vi "FinalSystem.vi"() -> ()   [LabVIEW 2017]
panel:
  in  "stop":bool
  out "Countdown":dbl
  out "x .or. y?":bool
  out "Frequency":dbl
  out "Ambulance":bool
  out "Fire":bool
  out "Police":bool
  out "Waveform Graph":dynamicdata(graph)
  out "Velocity":dbl
  out "Too Fast":bool
  out "Delta T":dbl
  out "Elapsed Time (s)":dbl
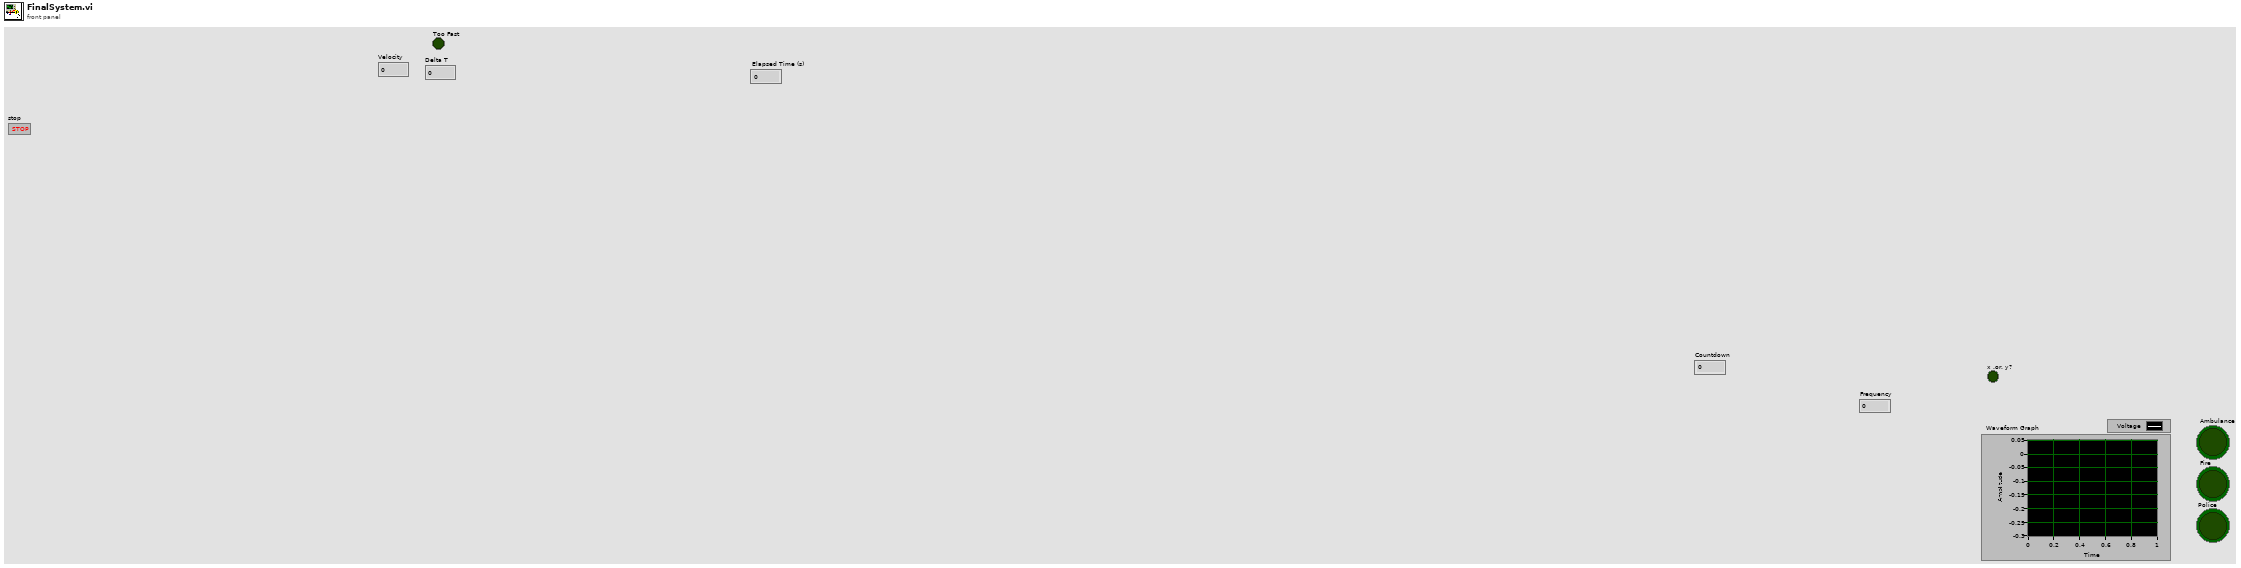
[diagram p1: front panel]
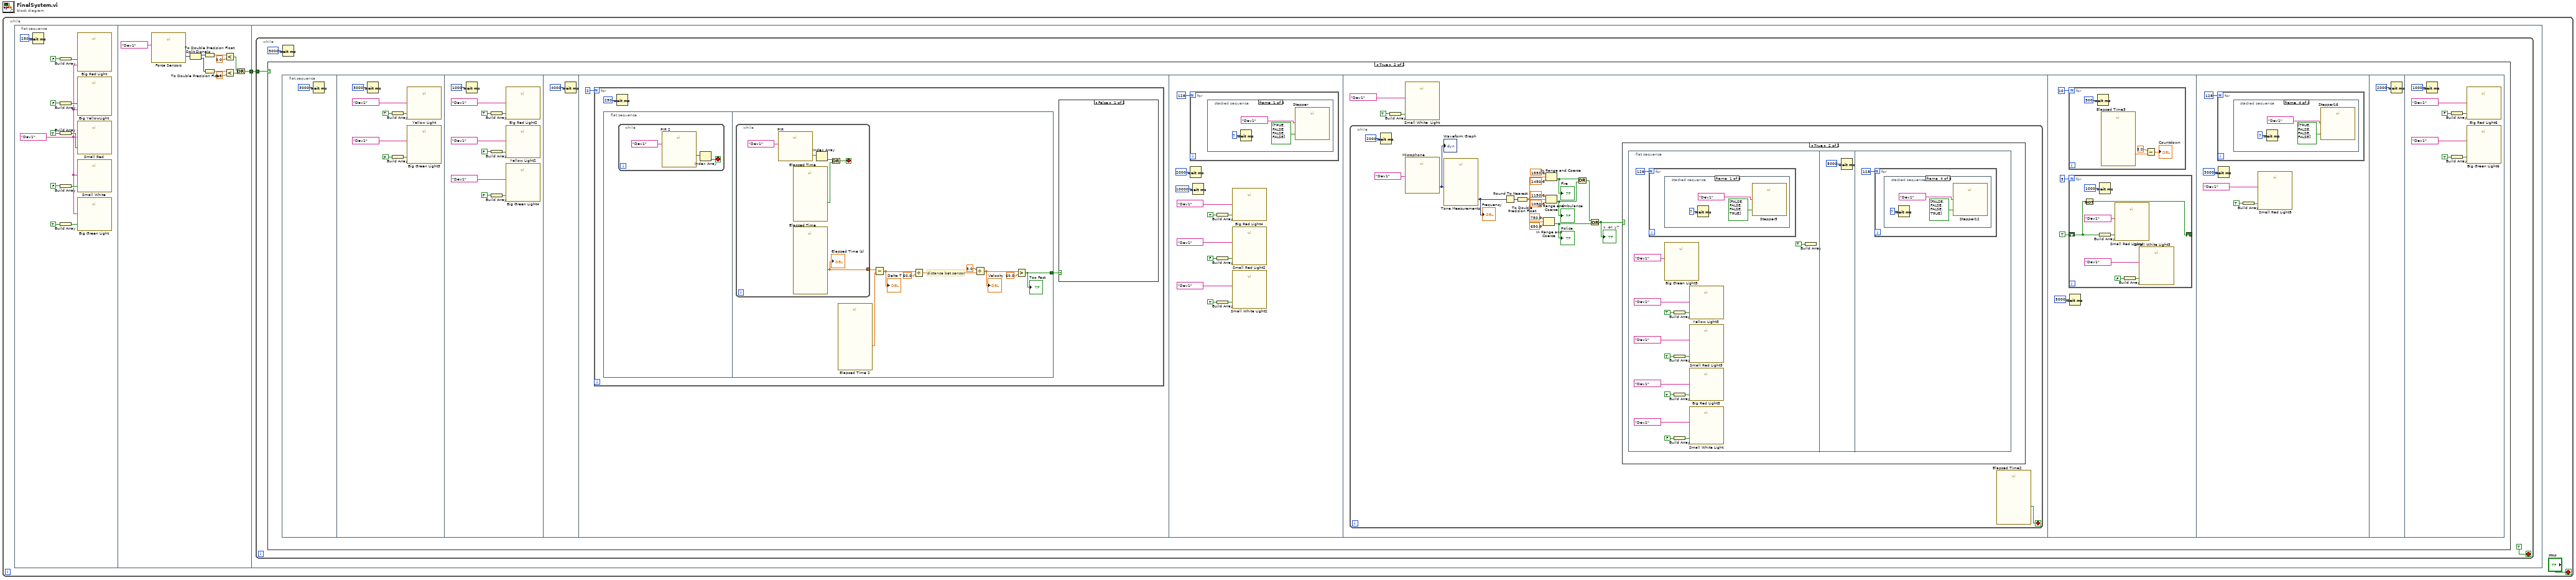
[diagram p0: block diagram]
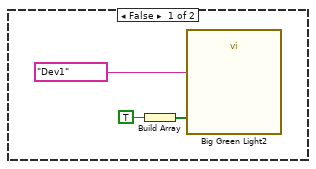
[diagram p2: hidden frame]
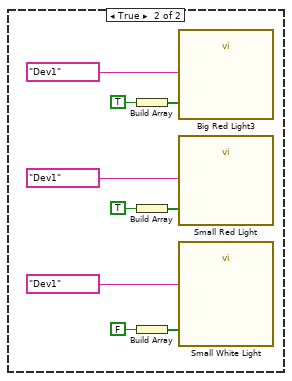
[diagram p3: hidden frame]
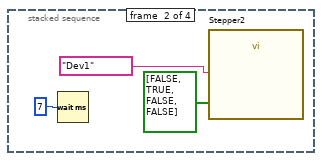
[diagram p4: hidden frame]
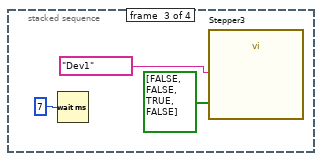
[diagram p5: hidden frame]
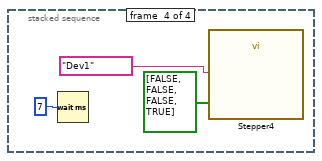
[diagram p6: hidden frame]
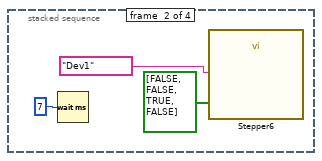
[diagram p8: hidden frame]
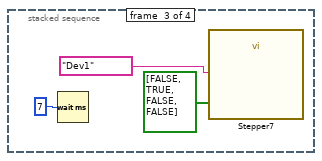
[diagram p9: hidden frame]
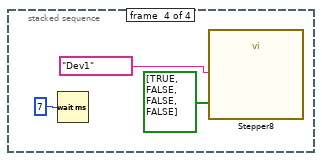
[diagram p10: hidden frame]
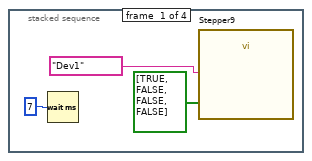
[diagram p11: hidden frame]
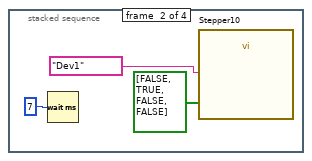
[diagram p12: hidden frame]
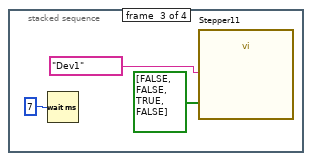
[diagram p13: hidden frame]
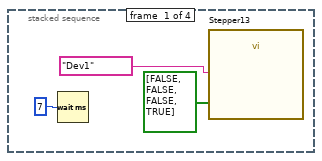
[diagram p14: hidden frame]
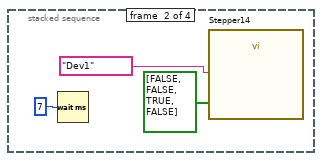
[diagram p15: hidden frame]
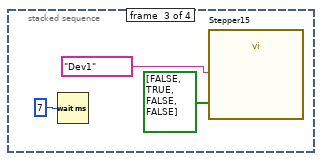
[diagram p16: hidden frame]
diagram:
  n1 = while {
    stop <- "stop" stop-if-true
    n2 = flat-sequence {
      tunnel: [w15] -> w2
      tunnel: w2 -> [w26]
      frame #0 {
        w3 = tag "Dev1" ("device name")
        n3 = Wait (ms)(milliseconds to wait=u32 250) -> ()  [unwired: 1 out]
        n4 = Build Array(FALSE) -> (w12:bool[])
        n5 = Build Array(FALSE) -> (w10:bool[])
        n6 = Build Array(TRUE) -> (w8:bool[])
        n7 = Build Array(FALSE) -> (w6:bool[])
        n8 = Build Array(TRUE) -> (w14:bool[])
        n9 = call "Big Red Light"("data"=w12, "device name"=w3) -> ()  [unwired: 16 in, 2 out]
        n10 = call "Big YellowLight"("data"=w10, "device name"=w3) -> ()  [unwired: 16 in, 2 out]
        n11 = call "Small Red"("data"=w8, "device name"=w3) -> ()  [unwired: 16 in, 2 out]
        n12 = call "Small White"("data"=w6, "device name"=w3) -> ()  [unwired: 16 in, 2 out]
        n13 = call "Big Green Light"("data"=w14, "device name"=w3) -> ()  [unwired: 16 in, 2 out]
      }
      frame #1 {
        n14 = call "Force Sensors"("device name"=tag "Dev1") -> ("data"=w18:dynamicdata)  [unwired: 16 in, 2 out]
        n15 = Split Signals(w18) -> (w17:dynamicdata, w16:dynamicdata)  [unwired: 2 in]
        n16 = To Double Precision Float(number=w17) -> (double precision float=w25:dbl)
        n17 = To Double Precision Float(number=w16) -> (double precision float=w22:dbl)
        n18 = Less?(x=w25, y=3.0) -> (x < y?=w19:bool)
        n19 = Less?(x=w22, y=3.0) -> (x < y?=w20:bool)
        n20 = Or(x=w19, y=w20) -> (x .or. y?=w15:bool)
      }
      frame #2 {
        n21 = while {
          tunnel: w26 -> [w28]
          stop <- TRUE stop-if-true
          n22 = case shown="True" w28 {
            frame False {
              n23 = Build Array(TRUE) -> (w32:bool[])
              n24 = call "Big Green Light2"("data"=w32, "device name"=tag "Dev1") -> ()  [unwired: 16 in, 2 out]
            }
            frame True {
              n25 = flat-sequence {
                frame #0 {
                  n26 = Wait (ms)(milliseconds to wait=u32 3000) -> ()  [unwired: 1 out]
                }
                frame #1 {
                  n27 = Wait (ms)(milliseconds to wait=u32 3000) -> ()  [unwired: 1 out]
                  n28 = Build Array(TRUE) -> (w40:bool[])
                  n29 = Build Array(FALSE) -> (w34:bool[])
                  n30 = call "Yellow Light"("data"=w40, "device name"=tag "Dev1") -> ()  [unwired: 16 in, 2 out]
                  n31 = call "Big Green Light3"("data"=w34, "device name"=tag "Dev1") -> ()  [unwired: 16 in, 2 out]
                }
                frame #2 {
                  n32 = Wait (ms)(milliseconds to wait=u32 1000) -> ()  [unwired: 1 out]
                  n33 = Build Array(TRUE) -> (w50:bool[])
                  n34 = Build Array(FALSE) -> (w49:bool[])
                  n35 = Build Array(FALSE) -> (w41:bool[])
                  n36 = call "Big Red Light2"("data"=w50, "device name"=tag "Dev1") -> ()  [unwired: 16 in, 2 out]
                  n37 = call "Yellow Light2"("data"=w49, "device name"=tag "Dev1") -> ()  [unwired: 16 in, 2 out]
                  n38 = call "Big Green Light4"("data"=w41, "device name"=tag "Dev1") -> ()  [unwired: 16 in, 2 out]
                }
                frame #3 {
                  n39 = Wait (ms)(milliseconds to wait=u32 4000) -> ()  [unwired: 1 out]
                }
                frame #4 {
                  n40 = for {
                    N: 2 -> [_]
                    n41 = flat-sequence {
                      tunnel: [w59] -> w53
                      frame #0 {
                        n42 = while {
                          stop <- w56 stop-if-true
                          n43 = call "PIR 2"("device name"=tag "Dev1") -> ("data"=w57:bool[])  [unwired: 16 in, 2 out]
                          n44 = Index Array(array=w57) -> (element=w56:bool)  [unwired: 1 in]
                        }
                      }
                      frame #1 {
                        # "distance bet sensor"
                        n45 = while {
                          tunnel: [w71] -> w61
                          stop <- w67 stop-if-true
                          n46 = call "PIR"("device name"=tag "Dev1") -> ("data"=w72:bool[])  [unwired: 16 in, 2 out]
                          n47 = call "Elapsed Time"() -> ("Time has Elapsed"=w68:bool)  [unwired: 12 in, 7 out]
                          n48 = call "Elapsed Time"() -> ("Elapsed Time (s)"=w71:dbl)  [unwired: 12 in, 7 out]
                          "Elapsed Time (s)" <- w71
                          n49 = Index Array(array=w72) -> (element=w69:bool)  [unwired: 1 in]
                          n50 = Or(x=w69, y=w68) -> (x .or. y?=w67:bool)
                        }
                        n51 = call "Elapsed Time 2"() -> ("Elapsed Time (s)"=w58:dbl)  [unwired: 12 in, 7 out]
                        n52 = Subtract(x=w61, y=w58) -> (x-y=w60:dbl)
                        "Delta T" <- w60
                        n53 = Divide(x=w60, y=60.0) -> (x/y=w63:dbl)
                        n54 = Divide(x=5.0, y=w63) -> (x/y=w65:dbl)
                        "Velocity" <- w65
                        n55 = Greater?(x=w65, y=60.0) -> (0:w59:bool)
                        "Too Fast" <- w59
                      }
                    }
                    n56 = Wait (ms)(milliseconds to wait=u32 250) -> ()  [unwired: 1 out]
                    n57 = case shown="False" w53 {
                      frame False {
                      }
                      frame True {
                        n58 = Build Array(TRUE) -> (w79:bool[])
                        n59 = Build Array(TRUE) -> (w80:bool[])
                        n60 = Build Array(FALSE) -> (w81:bool[])
                        n61 = call "Big Red Light3"("data"=w79, "device name"=tag "Dev1") -> ()  [unwired: 16 in, 2 out]
                        n62 = call "Small Red Light"("data"=w80, "device name"=tag "Dev1") -> ()  [unwired: 16 in, 2 out]
                        n63 = call "Small White Light"("data"=w81, "device name"=tag "Dev1") -> ()  [unwired: 16 in, 2 out]
                      }
                    }
                  }
                }
                frame #5 {
                  n64 = for {
                    N: 128 -> [_]
                    n65 = stacked-sequence {
                      frame #0 {
                        n66 = Wait (ms)(milliseconds to wait=u32 7) -> ()  [unwired: 1 out]
                        n67 = call "Stepper"("data"=bool[] [TRUE, FALSE, FALSE, FALSE], "device name"=tag "Dev1") -> ()  [unwired: 16 in, 2 out]
                      }
                      frame #1 {
                        n68 = Wait (ms)(milliseconds to wait=u32 7) -> ()  [unwired: 1 out]
                        n69 = call "Stepper2"("data"=bool[] [FALSE, TRUE, FALSE, FALSE], "device name"=tag "Dev1") -> ()  [unwired: 16 in, 2 out]
                      }
                      frame #2 {
                        n70 = Wait (ms)(milliseconds to wait=u32 7) -> ()  [unwired: 1 out]
                        n71 = call "Stepper3"("data"=bool[] [FALSE, FALSE, TRUE, FALSE], "device name"=tag "Dev1") -> ()  [unwired: 16 in, 2 out]
                      }
                      frame #3 {
                        n72 = Wait (ms)(milliseconds to wait=u32 7) -> ()  [unwired: 1 out]
                        n73 = call "Stepper4"("data"=bool[] [FALSE, FALSE, FALSE, TRUE], "device name"=tag "Dev1") -> ()  [unwired: 16 in, 2 out]
                      }
                    }
                  }
                  n74 = Wait (ms)(milliseconds to wait=u32 2000) -> ()  [unwired: 1 out]
                  n75 = Wait (ms)(milliseconds to wait=u32 10000) -> ()  [unwired: 1 out]
                  n76 = Build Array(TRUE) -> (w86:bool[])
                  n77 = Build Array(FALSE) -> (w91:bool[])
                  n78 = Build Array(TRUE) -> (w87:bool[])
                  n79 = call "Big Red Light4"("data"=w86, "device name"=tag "Dev1") -> ()  [unwired: 16 in, 2 out]
                  n80 = call "Small Red Light2"("data"=w91, "device name"=tag "Dev1") -> ()  [unwired: 16 in, 2 out]
                  n81 = call "Small White Light2"("data"=w87, "device name"=tag "Dev1") -> ()  [unwired: 16 in, 2 out]
                }
                frame #6 {
                  n82 = while {
                    stop <- w109 stop-if-true
                    n83 = Wait (ms)(milliseconds to wait=u32 2000) -> ()  [unwired: 1 out]
                    n84 = call "Microphone"("device name"=tag "Dev1") -> ("data"=w126:dynamicdata)  [unwired: 16 in, 2 out]
                    "Waveform Graph" <- w126
                    n85 = call "Tone Measurements"("Signals"=w126) -> ("Frequency"=w112:dynamicdata)  [unwired: 8 in, 2 out]
                    "Frequency" <- w112
                    n86 = Round To Nearest(number=w112) -> (nearest integer value=w111:dynamicdata)
                    n87 = To Double Precision Float(number=w111) -> (double precision float=w119:dbl)
                    n88 = In Range and Coerce(upper limit=750.0 ("y"), x=w119, lower limit=650.0 ("y")) -> (In Range?=w115:bool)  [unwired: 1 out]
                    "Police" <- w115
                    n89 = In Range and Coerce(upper limit=1550.0 ("y"), x=w119, lower limit=1450.0 ("y")) -> (In Range?=w117:bool)  [unwired: 1 out]
                    "Fire" <- w117
                    n90 = In Range and Coerce(upper limit=1150.0 ("y"), x=w119, lower limit=1050.0 ("y")) -> (In Range?=w116:bool)  [unwired: 1 out]
                    "Ambulance" <- w116
                    n91 = Or(x=w117, y=w116) -> (x .or. y?=w118:bool)
                    n92 = Or(x=w118, y=w115) -> (x .or. y?=w110:bool)
                    "x .or. y?" <- w110
                    n93 = case shown="True" w110 {
                      frame False {
                      }
                      frame True {
                        n94 = flat-sequence {
                          frame #0 {
                            n95 = for {
                              N: 128 -> [_]
                              n96 = stacked-sequence {
                                frame #0 {
                                n97 = Wait (ms)(milliseconds to wait=u32 7) -> ()  [unwired: 1 out]
                                n98 = call "Stepper5"("data"=bool[] [FALSE, FALSE, FALSE, TRUE], "device name"=tag "Dev1") -> ()  [unwired: 16 in, 2 out]
                                }
                                frame #1 {
                                n99 = Wait (ms)(milliseconds to wait=u32 7) -> ()  [unwired: 1 out]
                                n100 = call "Stepper6"("data"=bool[] [FALSE, FALSE, TRUE, FALSE], "device name"=tag "Dev1") -> ()  [unwired: 16 in, 2 out]
                                }
                                frame #2 {
                                n101 = Wait (ms)(milliseconds to wait=u32 7) -> ()  [unwired: 1 out]
                                n102 = call "Stepper7"("data"=bool[] [FALSE, TRUE, FALSE, FALSE], "device name"=tag "Dev1") -> ()  [unwired: 16 in, 2 out]
                                }
                                frame #3 {
                                n103 = Wait (ms)(milliseconds to wait=u32 7) -> ()  [unwired: 1 out]
                                n104 = call "Stepper8"("data"=bool[] [TRUE, FALSE, FALSE, FALSE], "device name"=tag "Dev1") -> ()  [unwired: 16 in, 2 out]
                                }
                              }
                            }
                            n105 = call "Big Green Light5"("device name"=tag "Dev1") -> ()  [unwired: 17 in, 2 out]
                            n106 = Build Array(TRUE) -> (w140:bool[])
                            n107 = Build Array(TRUE) -> (w130:bool[])
                            n108 = Build Array(TRUE) -> (w141:bool[])
                            n109 = Build Array(FALSE) -> (w127:bool[])
                            n110 = call "Yellow Light3"("data"=w140, "device name"=tag "Dev1") -> ()  [unwired: 16 in, 2 out]
                            n111 = call "Small Red Light3"("data"=w130, "device name"=tag "Dev1") -> ()  [unwired: 16 in, 2 out]
                            n112 = call "Big Red Light5"("data"=w141, "device name"=tag "Dev1") -> ()  [unwired: 16 in, 2 out]
                            n113 = call "Small White Light"("data"=w127, "device name"=tag "Dev1") -> ()  [unwired: 16 in, 2 out]
                            n114 = Build Array(TRUE) -> ()  [unwired: 1 out]
                          }
                          frame #1 {
                            n115 = Wait (ms)(milliseconds to wait=u32 5000) -> ()  [unwired: 1 out]
                          }
                          frame #2 {
                            n116 = for {
                              N: 128 -> [_]
                              n117 = stacked-sequence {
                                frame #0 {
                                n118 = Wait (ms)(milliseconds to wait=u32 7) -> ()  [unwired: 1 out]
                                n119 = call "Stepper9"("data"=bool[] [TRUE, FALSE, FALSE, FALSE], "device name"=tag "Dev1") -> ()  [unwired: 16 in, 2 out]
                                }
                                frame #1 {
                                n120 = Wait (ms)(milliseconds to wait=u32 7) -> ()  [unwired: 1 out]
                                n121 = call "Stepper10"("data"=bool[] [FALSE, TRUE, FALSE, FALSE], "device name"=tag "Dev1") -> ()  [unwired: 16 in, 2 out]
                                }
                                frame #2 {
                                n122 = Wait (ms)(milliseconds to wait=u32 7) -> ()  [unwired: 1 out]
                                n123 = call "Stepper11"("data"=bool[] [FALSE, FALSE, TRUE, FALSE], "device name"=tag "Dev1") -> ()  [unwired: 16 in, 2 out]
                                }
                                frame #3 {
                                n124 = Wait (ms)(milliseconds to wait=u32 7) -> ()  [unwired: 1 out]
                                n125 = call "Stepper12"("data"=bool[] [FALSE, FALSE, FALSE, TRUE], "device name"=tag "Dev1") -> ()  [unwired: 16 in, 2 out]
                                }
                              }
                            }
                          }
                        }
                      }
                    }
                    n126 = call "Elapsed Time2"() -> ("Time has Elapsed"=w109:bool)  [unwired: 12 in, 7 out]
                  }
                  n127 = Build Array(TRUE) -> (w108:bool[])
                  n128 = call "Small White  Light"("data"=w108, "device name"=tag "Dev1") -> ()  [unwired: 16 in, 2 out]
                }
                frame #7 {
                  n129 = for {
                    N: 10 -> [_]
                    n130 = Wait (ms)(milliseconds to wait=u32 500) -> ()  [unwired: 1 out]
                    n131 = call "Elapsed Time3"() -> ("Elapsed Time (s)"=w182:dbl)  [unwired: 12 in, 7 out]
                    n132 = Subtract(x=5.0, y=w182) -> (x-y=→"Countdown":dbl)
                  }
                  n133 = for {
                    N: 5 -> [_]
                    shift-right: [w179] -> _
                    shift-left: TRUE -> [w178]
                    n134 = Not(x=w178) -> (.not. x?=w179:bool)
                    n135 = Wait (ms)(milliseconds to wait=u32 1000) -> ()  [unwired: 1 out]
                    n136 = Build Array(w178) -> (w177:bool[])
                    n137 = call "Small Red Light4"("data"=w177, "device name"=tag "Dev1") -> ()  [unwired: 16 in, 2 out]
                    n138 = Build Array(FALSE) -> (w175:bool[])
                    n139 = call "Small White Light3"("data"=w175, "device name"=tag "Dev1") -> ()  [unwired: 16 in, 2 out]
                  }
                  n140 = Wait (ms)(milliseconds to wait=u32 5000) -> ()  [unwired: 1 out]
                }
                frame #8 {
                  n141 = for {
                    N: 128 -> [_]
                    n142 = stacked-sequence {
                      frame #0 {
                        n143 = Wait (ms)(milliseconds to wait=u32 7) -> ()  [unwired: 1 out]
                        n144 = call "Stepper13"("data"=bool[] [FALSE, FALSE, FALSE, TRUE], "device name"=tag "Dev1") -> ()  [unwired: 16 in, 2 out]
                      }
                      frame #1 {
                        n145 = Wait (ms)(milliseconds to wait=u32 7) -> ()  [unwired: 1 out]
                        n146 = call "Stepper14"("data"=bool[] [FALSE, FALSE, TRUE, FALSE], "device name"=tag "Dev1") -> ()  [unwired: 16 in, 2 out]
                      }
                      frame #2 {
                        n147 = Wait (ms)(milliseconds to wait=u32 7) -> ()  [unwired: 1 out]
                        n148 = call "Stepper15"("data"=bool[] [FALSE, TRUE, FALSE, FALSE], "device name"=tag "Dev1") -> ()  [unwired: 16 in, 2 out]
                      }
                      frame #3 {
                        n149 = Wait (ms)(milliseconds to wait=u32 7) -> ()  [unwired: 1 out]
                        n150 = call "Stepper16"("data"=bool[] [TRUE, FALSE, FALSE, FALSE], "device name"=tag "Dev1") -> ()  [unwired: 16 in, 2 out]
                      }
                    }
                  }
                  n151 = Wait (ms)(milliseconds to wait=u32 3000) -> ()  [unwired: 1 out]
                  n152 = Build Array(TRUE) -> (w188:bool[])
                  n153 = call "Small Red Light5"("data"=w188, "device name"=tag "Dev1") -> ()  [unwired: 16 in, 2 out]
                }
                frame #9 {
                  n154 = Wait (ms)(milliseconds to wait=u32 2000) -> ()  [unwired: 1 out]
                }
                frame #10 {
                  n155 = Wait (ms)(milliseconds to wait=u32 1000) -> ()  [unwired: 1 out]
                  n156 = Build Array(FALSE) -> (w207:bool[])
                  n157 = Build Array(TRUE) -> (w208:bool[])
                  n158 = call "Big Red Light6"("data"=w207, "device name"=tag "Dev1") -> ()  [unwired: 16 in, 2 out]
                  n159 = call "Big Green Light6"("data"=w208, "device name"=tag "Dev1") -> ()  [unwired: 16 in, 2 out]
                }
              }
            }
          }
          n160 = Wait (ms)(milliseconds to wait=u32 5000) -> ()  [unwired: 1 out]
        }
      }
    }
  }
